vi "ReversedEngineering_GetClassAttrubutes.vi"(1 "Path":path, 5 "error in (no error)":errorcluster) -> (15 "attributeInfo":T1[](array[typedef]), 19 "error out":errorcluster)   [LabVIEW 2016]
uses:
  <resource>/Framework/Providers/Open_GDS/UML/ReversedEngineering/ReversedEngineering AttributeInfoType.ctl
  <resource>/Framework/Providers/Open_GDS/ClassProviders/Common/CommonVIs/CommonVIs_AttributeDataType.ctl
  <resource>/Framework/Providers/Open_GDS/UML/UMLEditor/UMLEditor_VisibilityType.ctl
panel:
  out "Owning VI":refnum<vi>
  out "Callees' Names":string[](array[string])
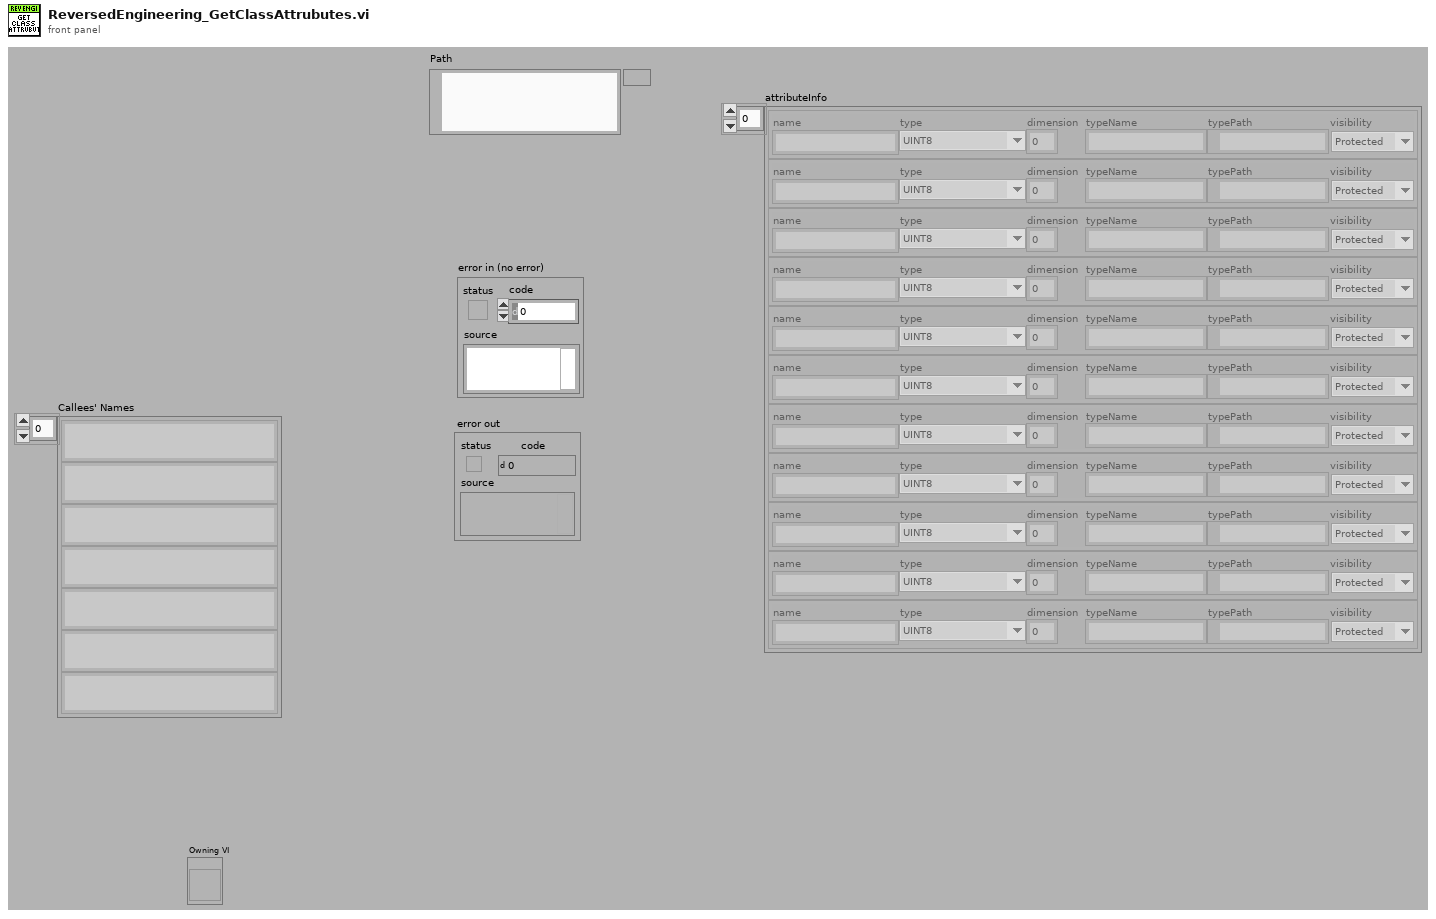
[diagram p1: front panel]
types:
  T1 = typedef "ReversedEngineering AttributeInfoType.ctl" = cluster{"name":string, "type":T2, "dimension":i32, "typeName":string, "typePath":path, "visibility":T3}
  T2 = typedef "CommonVIs_AttributeDataType.ctl" = enum16{"UINT8", "INT8", "UINT16", "INT16", "UINT32", "INT32", "UINT64", "INT64", "SGL", "DBL", "EXT", "CSG", "CDB", "CXT", "TimeStamp", "STRING", "PATH", "BOOL", "ENUM", "RefNum", "VIRefNum", "LabVIEW Class", "Cluster", "Variant", "TypeDef", "Waveform", "LabVIEW Object", "Other", "void"}
  T3 = typedef "UMLEditor_VisibilityType.ctl" = enum16{"Public", "Private", "Protected"}
  T4 = cluster{"name":string, "typeDesc":i16[], "dim":i32}[]
  T5 = cluster{"Label.Text":string, "typeDesc":i16[], "index":i32}[]
  T6 = cluster{"Label.Text":string, "typeDesc":i16[], "dim":i32}[]
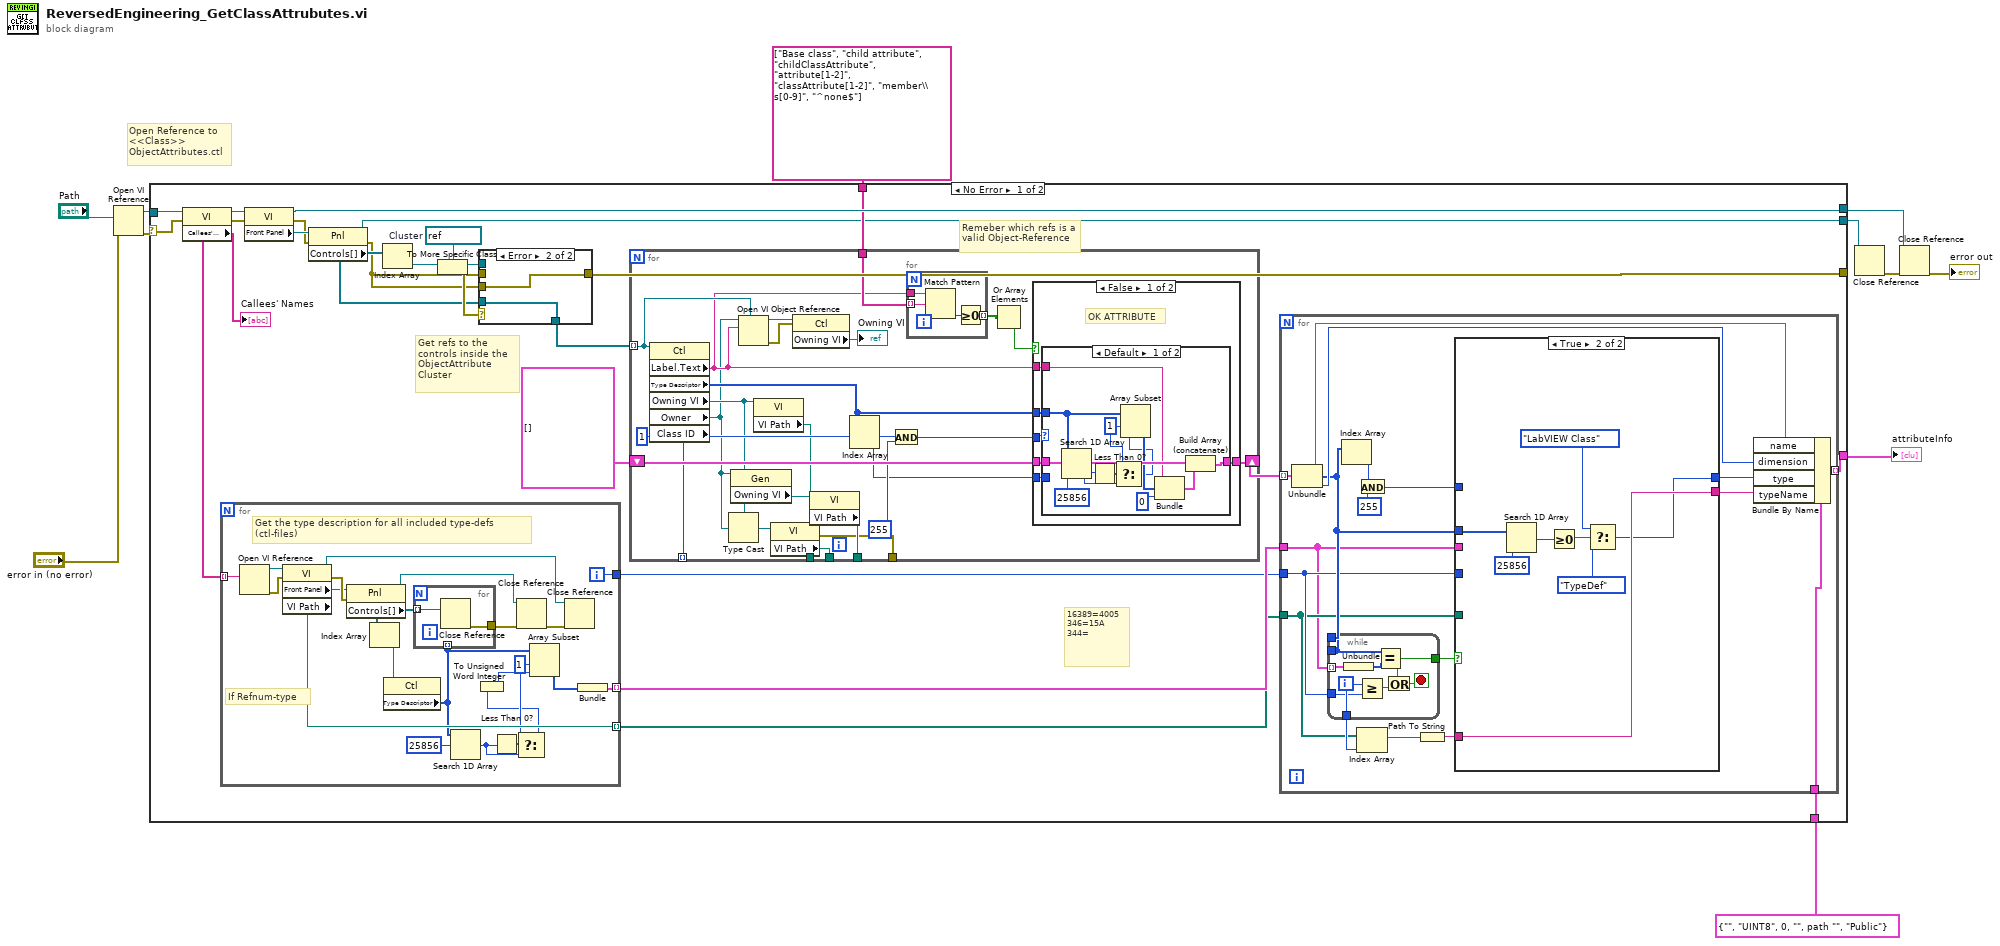
[diagram p0: block diagram]
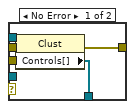
[diagram p2: hidden frame]
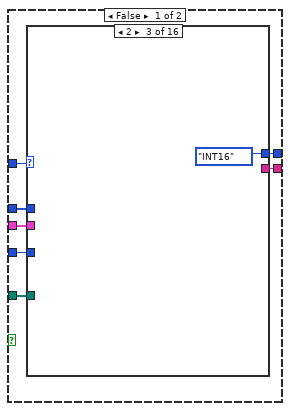
[diagram p3: hidden frame]
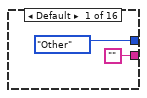
[diagram p4: hidden frame]
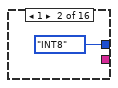
[diagram p5: hidden frame]
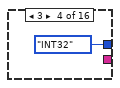
[diagram p6: hidden frame]
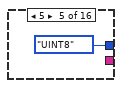
[diagram p7: hidden frame]
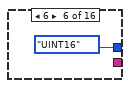
[diagram p8: hidden frame]
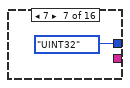
[diagram p9: hidden frame]
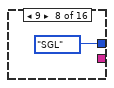
[diagram p10: hidden frame]
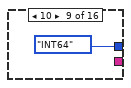
[diagram p11: hidden frame]
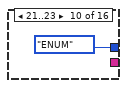
[diagram p12: hidden frame]
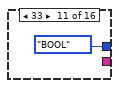
[diagram p13: hidden frame]
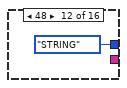
[diagram p14: hidden frame]
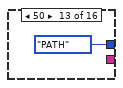
[diagram p15: hidden frame]
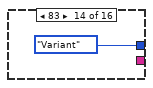
[diagram p16: hidden frame]
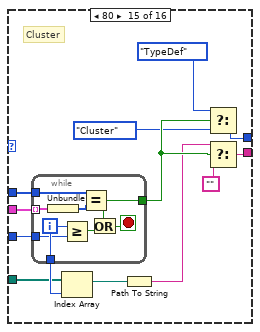
[diagram p17: hidden frame]
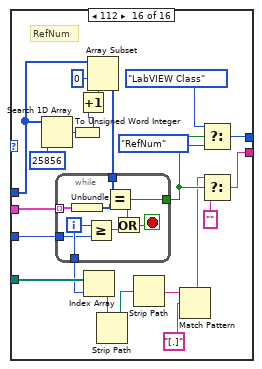
[diagram p18: hidden frame]
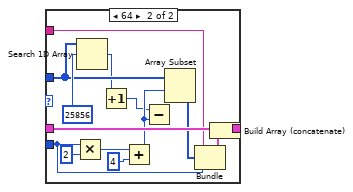
[diagram p19: hidden frame]
diagram:
  # "Open Reference to <<Class>> ObjectAttributes.ctl"
  n1 = Open VI Reference(vi path="Path", error in (no error)="error in (no error)") -> (vi reference=w10:refnum<vi>, error out=w6:errorcluster)  [unwired: 4 out]
  n2 = case shown="No Error" w6 {
    selector: w6 -> [w21 w237]
    tunnel: w10 -> [w36 w236]
    tunnel: [w27 w236] -> w9
    tunnel: [w23 w237] -> _
    tunnel: [w18 _] -> w5
    tunnel: string[] ["Base class", "child attribute", "childClassAttribute", "attribute[1-2]", "classAttribute[1-2]", "member\\s[0-9]", "^none$"] -> [w17 _]
    tunnel: [w16 _] -> w2
    tunnel: T1 {"name"="", "type"=enum."UINT8", "dimension"=0, "typeName"="", "typePath"=path "", "visibility"=enum."Public"} ("attributeInfoType") -> [w15 _]
    frame No Error {
      w31 = refnum<vi> refnum  # Cluster
      # "16389=4005\n346=15A\n344="
      # "Remeber which refs is a valid Object-Reference"
      # "Get refs to the controls inside the ObjectAttribute Cluster"
      n3 = property class="VI"(reference=w36, error in=w21) -> (reference out=w35:refnum<vi>, error out=w34:errorcluster, "Callees' Names"=w26:string[])
      "Callees' Names" <- w26
      n4 = for {
        tunnel: w26 -> [w64] mode=indexing
        tunnel: [w58] -> w25 mode=indexing
        tunnel: [w57] -> w19 mode=indexing
        tunnel: [w56] -> w24
        i -> [w56]
        w46 = 1 ("index")
        # "If Refnum-type"
        # "Get the type description for all included type-defs (ctl-files)"
        n5 = Open VI Reference(vi path=w64) -> (vi reference=w61:refnum<vi>, error out=w60:errorcluster)  [unwired: 1 in, 4 out]
        n6 = property class="VI"(reference=w61, error in=w60) -> (reference out=w48:refnum<vi>, error out=w63:errorcluster, "Front Panel"=w62:refnum<vi>, "VI Path"=w57:path)
        n7 = property class="Pnl"(reference=w62, error in=w63) -> (reference out=w50:refnum<vi>, "Controls[]"=w52:refnum<vi>[])  [unwired: 1 out]
        n8 = Index Array(array=w52) -> (element=w59:refnum<vi>)  [unwired: 1 in]
        n9 = property class="Ctl"(reference=w59) -> ("Type Descriptor"=w43:i16[])  [unwired: 1 in, 2 out]
        n10 = for {
          tunnel: w52 -> [w66] mode=indexing
          tunnel: [w65] -> w51
          tunnel: w43 -> [_] mode=indexing
          n11 = Close Reference(reference=w66) -> (error out=w65:errorcluster)  [unwired: 1 in]
        }
        n12 = Search 1D Array(1D array=w43, element=i16 25856) -> (index of element=w45:i32)  [unwired: 1 out]
        n13 = Less Than 0?(x=w45) -> (x < 0?=w47:bool)
        n14 = Close Reference(reference=w50, error in (no error)=w51) -> (error out=w49:errorcluster)
        n15 = Select(t=w46, s=w47, f=w45) -> (s? t:f=w44:i32)
        n16 = To Unsigned Word Integer(number=w44) -> (unsigned 16bit integer=w53:u16)
        n17 = Array Subset(array=w43, index=w46, length=w53) -> (w55:i16[])
        n18 = Close Reference(reference=w48, error in (no error)=w49) -> ()  [unwired: 1 out]
        n19 = Bundle(w55) -> (w58:cluster{i16[]})  [unwired: 1 in]
      }
      n20 = property class="VI"(reference=w35, error in=w34) -> (reference out=w27:refnum<vi>, error out=w28:errorcluster, "Front Panel"=w33:refnum<vi>)
      n21 = property class="Pnl"(reference=w33, error in=w28) -> (reference out=w16:refnum<vi>, error out=w12:errorcluster, "Controls[]"=w13:refnum<vi>[])
      n22 = Index Array(array=w13) -> (element=w32:refnum<vi>)  [unwired: 1 in]
      n23 = To More Specific Class(target class=w31, reference=w32) -> (specific class reference=w30:refnum<vi>, error out=w14:errorcluster)  [unwired: 1 in]
      n24 = case shown="Error" w14 {
        tunnel: w30 -> [w40 _]
        tunnel: [w39 w42] -> w29
        tunnel: w12 -> [w38 _]
        tunnel: [w37 w41] -> w23
        tunnel: w13 -> [_ w42]
        tunnel: w12 -> [_ w41]
        frame No Error {
          n25 = property class="Clust"(reference=w40, error in=w38) -> (error out=w37:errorcluster, "Controls[]"=w39:refnum<vi>[])  [unwired: 1 out]
        }
        frame Error {
        }
      }
      n26 = for {
        tunnel: w29 -> [w177] mode=indexing
        shift-right: [w197] -> w20
        shift-left: T4 [] -> [w198]
        tunnel: w17 -> [w188]
        tunnel: [w186] -> _
        tunnel: [w185] -> _
        tunnel: [w182] -> _
        tunnel: [w181] -> _
        tunnel: [w174] -> _ mode=indexing
        n27 = property class="Ctl"(reference=w177) -> ("Label.Text"=w176:string, "Type Descriptor"=w192:i16[], "Owning VI"=w184:refnum<vi>, "Owner"=w175:refnum<vi>, "Class ID"=w174:u32)  [unwired: 1 in, 2 out]
        n28 = Type Cast(type=w184, x=w175) -> (*(type *) &x=w183:refnum<vi>)
        n29 = property class="Gen"(reference=w175) -> ("Owning VI"=w187:refnum<vi>)  [unwired: 1 in, 2 out]
        n30 = Open VI Object Reference(7:w177, 10:w176, 11:w175) -> (0:w179:errorcluster, 3:w180:refnum<vi>)  [unwired: 1 in]
        n31 = property class="VI"(reference=w184) -> ("VI Path"=w186:path)  [unwired: 1 in, 2 out]
        n32 = property class="VI"(reference=w183) -> (error out=w182:errorcluster, "VI Path"=w181:path)  [unwired: 1 in, 1 out]
        n33 = property class="Ctl"(reference=w180, error in=w179) -> ("Owning VI"=→"Owning VI":refnum<vi>)  [unwired: 2 out]
        n34 = property class="VI"(reference=w187) -> ("VI Path"=w185:path)  [unwired: 1 in, 2 out]
        n35 = Index Array(array=w192, index #1=1 ("index")) -> (element #1=w195:i16, element #2=w191:i16)  [unwired: 1 in]
        n36 = And(x=w195, y=i16 255) -> (x .and. y?=w193:i16)
        n37 = for {
          tunnel: [w201] -> w190 mode=indexing
          tunnel: w176 -> [w200]
          tunnel: w188 -> [w199] mode=indexing
          n38 = Match Pattern(string=w200, regular expression=w199) -> (offset past match=w202:i32)  [unwired: 4 out]
          n39 = Greater Or Equal To 0?(x=w202) -> (x >= 0?=w201:bool)
        }
        n40 = Or Array Elements(Boolean array=w190) -> (logical OR=w189:bool)
        n41 = case shown="False" w189 {
          tunnel: w198 -> [w208 w235]
          tunnel: [w207 w235] -> w197
          tunnel: w193 -> [w206 _]
          tunnel: w192 -> [w205 _]
          tunnel: w191 -> [w204 _]
          tunnel: w176 -> [w203 _]
          frame False {
            # "OK ATTRIBUTE"
            n42 = case shown="Default" w206 {
              tunnel: w208 -> [w220 w234]
              tunnel: [w219 w233] -> w207
              tunnel: w205 -> [w217 w228]
              tunnel: w204 -> [_ w224]
              tunnel: w203 -> [w214 w222]
              frame Default {
                w209 = 1 ("index")
                n43 = Search 1D Array(1D array=w217, element=i16 25856) -> (index of element=w210:i32)  [unwired: 1 out]
                n44 = Less Than 0?(x=w210) -> (x < 0?=w213:bool)
                n45 = Select(t=w209, s=w213, f=w210) -> (s? t:f=w212:i32)
                n46 = Array Subset(array=w217, index=w209, length=w212) -> (w215:i16[])
                n47 = Bundle("Label.Text"=w214, w215, "index"=0) -> (w216:cluster{"Label.Text":string, i16[], "index":i32})  [unwired: 1 out]
                n48 = Build Array (concatenate)(w220, w216) -> (w219:T5)
              }
              frame 64 {
                n49 = Multiply(x=w224, y=i16 2) -> (x*y=w231:i16)
                n50 = Search 1D Array(1D array=w228, element=i16 25856) -> (index of element=w227:i32)  [unwired: 1 out]
                n51 = Increment(x=w227) -> (x+1=w225:i32)
                n52 = Add(x=w231, y=i16 4) -> (x+y=w226:i16)
                n53 = Subtract(x=w225, y=w226) -> ()  [unwired: 1 out]
                n54 = Array Subset(array=w228, index=w226) -> (w223:i16[])  [unwired: 1 in]
                n55 = Bundle("Label.Text"=w222, w223, w224) -> (w221:cluster{"Label.Text":string, i16[], i16})  [unwired: 1 out]
                n56 = Build Array (concatenate)(w234, w221) -> (w233:T6)
              }
            }
          }
          frame True {
            # "IGNORE SINCE IT IS A DEFAULT\nATTRIBUTE THAT HAS TO EXIST"
          }
        }
      }
      n57 = for {
        tunnel: w20 -> [w84] mode=indexing
        tunnel: w25 -> [w68]
        tunnel: w24 -> [w72]
        tunnel: w15 -> [w80]
        tunnel: w19 -> [w71]
        tunnel: [w76] -> w18 mode=indexing
        n58 = Unbundle(w84) -> ("name"=w79:string, "typeDesc"=w73:i16[], "dim"=w78:i32)
        n59 = while {
          tunnel: w68 -> [w173] mode=indexing
          tunnel: [w166] -> _
          tunnel: w72 -> [w171]
          tunnel: [w172] -> w74
          tunnel: [w170] -> w70
          tunnel: w73 -> [w166]
          i -> [w172]
          stop <- w168 stop-if-true
          n60 = Unbundle(w173) -> (w167:i16[])
          n61 = Greater Or Equal?(x=w172, y=w171) -> (x >= y?=w169:bool)
          n62 = Equal?(x=w166, y=w167) -> (x = y?=w170:bool)
          n63 = Or(x=w170, y=w169) -> (x .or. y?=w168:bool)
        }
        n64 = Index Array(array=w73) -> (element=w82:i16)  [unwired: 1 in]
        n65 = Index Array(array=w71, index=w74) -> (element=w75:path)
        n66 = And(x=w82, y=i16 255) -> (x .and. y?=w81:i16)
        n67 = Path To String(path=w75) -> (string=w69:string)
        n68 = case shown="True" w70 {
          tunnel: w68 -> [w91 _]
          tunnel: w81 -> [w90 _]
          tunnel: [w89 w160] -> w67
          tunnel: [w88 w165] -> w77
          tunnel: w73 -> [w87 w163]
          tunnel: w72 -> [w86 _]
          tunnel: w71 -> [w85 _]
          tunnel: w69 -> [_ w165]
          frame False {
            n69 = case shown="2" w90 {
              tunnel: w91 -> [_ _ _ _ _ _ _ _ _ _ _ _ _ _ w119 w142]
              tunnel: w86 -> [_ _ _ _ _ _ _ _ _ _ _ _ _ _ w118 w133]
              tunnel: w87 -> [_ _ _ _ _ _ _ _ _ _ _ _ _ _ w117 w145]
              tunnel: [CommonVIs_AttributeDataType."Other" ("type") CommonVIs_AttributeDataType."INT8" ("type") CommonVIs_AttributeDataType."INT16" ("type") CommonVIs_AttributeDataType."INT32" ("type") CommonVIs_AttributeDataType."UINT8" ("type") CommonVIs_AttributeDataType."UINT16" ("type") CommonVIs_AttributeDataType."UINT32" ("type") CommonVIs_AttributeDataType."SGL" ("type") CommonVIs_AttributeDataType."INT64" ("type") CommonVIs_AttributeDataType."ENUM" ("type") CommonVIs_AttributeDataType."BOOL" ("type") CommonVIs_AttributeDataType."STRING" ("type") CommonVIs_AttributeDataType."PATH" ("type") CommonVIs_AttributeDataType."Variant" ("type") w112 w138] -> w89
              tunnel: ["" _ _ _ _ _ _ _ _ _ _ _ _ _ w115 w135] -> w88
              tunnel: w85 -> [_ _ _ _ _ _ _ _ _ _ _ _ _ _ w113 w140]
              frame Default {
              }
              frame 1 {
              }
              frame 2 {
              }
              frame 3 {
              }
              frame 5 {
              }
              frame 6 {
              }
              frame 7 {
              }
              frame 9 {
              }
              frame 10 {
              }
              frame 21..23 {
              }
              frame 33 {
              }
              frame 48 {
              }
              frame 50 {
              }
              frame 83 {
              }
              frame 80 {
                # "Cluster"
                n70 = while {
                  tunnel: w119 -> [w127] mode=indexing
                  tunnel: w117 -> [w126]
                  tunnel: w118 -> [w124]
                  tunnel: [w125] -> w114
                  tunnel: [w123] -> w111
                  i -> [w125]
                  stop <- w121 stop-if-true
                  n71 = Unbundle(w127) -> (w120:i16[])
                  n72 = Greater Or Equal?(x=w125, y=w124) -> (x >= y?=w122:bool)
                  n73 = Equal?(x=w126, y=w120) -> (x = y?=w123:bool)
                  n74 = Or(x=w123, y=w122) -> (x .or. y?=w121:bool)
                }
                n75 = Index Array(array=w113, index=w114) -> (element=w110:path)
                n76 = Path To String(path=w110) -> (string=w109:string)
                n77 = Select(t=CommonVIs_AttributeDataType."TypeDef" ("type"), s=w111, f=CommonVIs_AttributeDataType."Cluster" ("type")) -> (s? t:f=w112:T2)
                n78 = Select(t=w109, s=w111, f="") -> (s? t:f=w115:string)
              }
              frame 112 {
                # "RefNum"
                n79 = Search 1D Array(1D array=w145, element=i16 25856) -> (index of element=w147:i32)  [unwired: 1 out]
                n80 = To Unsigned Word Integer(number=w147) -> (unsigned 16bit integer=w146:u16)
                n81 = Increment(x=w146) -> (x+1=w132:u16)
                n82 = Array Subset(array=w145, index=0, length=w132) -> (w141:i16[])
                n83 = while {
                  tunnel: w142 -> [w157] mode=indexing
                  tunnel: [w156] -> w139
                  tunnel: [w155] -> w137
                  tunnel: w141 -> [w151]
                  tunnel: w133 -> [w150]
                  i -> [w156]
                  stop <- w153 stop-if-true
                  n84 = Unbundle(w157) -> (w152:i16[])
                  n85 = Greater Or Equal?(x=w156, y=w150) -> (x >= y?=w154:bool)
                  n86 = Equal?(x=w151, y=w152) -> (x = y?=w155:bool)
                  n87 = Or(x=w155, y=w154) -> (x .or. y?=w153:bool)
                }
                n88 = Index Array(array=w140, index=w139) -> (element=w144:path)
                n89 = Strip Path(path=w144) -> (stripped path=w131:path)  [unwired: 1 out]
                n90 = Strip Path(path=w131) -> (name=w130:string)  [unwired: 1 out]
                n91 = Match Pattern(string=w130, regular expression="[.]") -> (before substring=w136:string)  [unwired: 4 out]
                n92 = Select(t=CommonVIs_AttributeDataType."LabVIEW Class" ("type"), s=w137, f=CommonVIs_AttributeDataType."RefNum" ("type")) -> (s? t:f=w138:T2)
                n93 = Select(t=w136, s=w137, f="") -> (s? t:f=w135:string)
              }
            }
          }
          frame True {
            n94 = Search 1D Array(1D array=w163, element=i16 25856) -> (index of element=w162:i32)  [unwired: 1 out]
            n95 = Greater Or Equal To 0?(x=w162) -> (x >= 0?=w161:bool)
            n96 = Select(t=CommonVIs_AttributeDataType."LabVIEW Class" ("type"), s=w161, f=CommonVIs_AttributeDataType."TypeDef" ("type")) -> (s? t:f=w160:T2)
          }
        }
        n97 = Bundle By Name(cluster=w80, "name"=w79, "dimension"=w78, "type"=w67, "typeName"=w77) -> (w76:T1)
      }
    }
    frame Error {
    }
  }
  "attributeInfo" <- w5
  n98 = Close Reference(reference=w2) -> (error out=w3:errorcluster)  [unwired: 1 in]
  n99 = Close Reference(reference=w9, error in (no error)=w3) -> (error out=→"error out":errorcluster)
